vi "saturation_fxp.vi"(7 "uMax":fxp<+/-,32,6>, 10 "signal_in":fxp<+/-,32,6>) -> (0 "has_saturated":bool, 2 "signal_out (saturated)":fxp<+/-,32,6>)   [LabVIEW 2017]
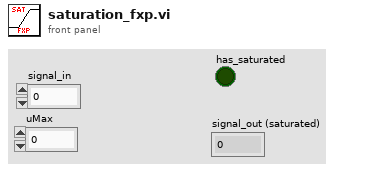
[diagram p1: front panel]
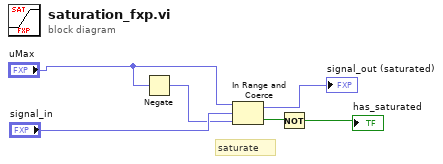
[diagram p0: block diagram]
diagram:
  # "saturate"
  n1 = Negate(x="uMax") -> (-x=w2:fxp<+/-,18,5>)
  n2 = In Range and Coerce(upper limit="uMax", x="signal_in", lower limit=w2) -> (coerced(x)=→"signal_out (saturated)":fxp<+/-,32,6>, In Range?=w5:bool)
  n3 = Not(x=w5) -> (.not. x?=→"has_saturated":bool)
